vi "Teleop.vi"(10 "Match Info":T1={"Autonomous Elapsed Seconds"=0.0, "TeleOp Elapsed Seconds"=0.0, "Disabled Elapsed Seconds"=0.0, "Visited Autonomous"=FALSE, "Visited TeleOp"=FALSE, "Visited Disabled"=FALSE, "Autonomous Settings"={"Autonomous Style"=enum."Independent", "VI Refnum"=refnum}}, 11 "Call Context":T2) -> ()   [LabVIEW 2014]
doc: "This VI is called for each TeleOp packet received from the DS where the robot is not disabled. It is often used to read from the joysticks and update I/O or to update setpoints for timed control loops. It should complete and return within 20 milliseconds or it may miss DS packets."
uses:
  <vilib>/Rock Robotics/WPI/DriverStation/WPI_DriverStationDerivedRobotMode.ctl
  <vilib>/Rock Robotics/WPI/DriverStation/WPI_DriverStationMatch Info.ctl
  Robot Global Data.vi
  <vilib>/Rock Robotics/WPI/Joystick/WPI_JoystickGetSetRefNum.vi
  <vilib>/Rock Robotics/WPI/RobotDrive/WPI_RobotDriveGetSetRefNum.vi
panel:
  out "toggle on/off 2":bool=TRUE
  in  "toggle on/off internal 2":bool=TRUE
  in  "last switch 2":bool
  out "axis 1 (x) 2":dbl
  out "axis 2 (y) 2":dbl
  out "toggle on/off":bool=TRUE
  in  "toggle on/off internal":bool=TRUE
  in  "last switch":bool
  out "axis 1 (x)":dbl
  out "axis 2 (y)":dbl
  out "Numeric 1":dbl(slide) scale=0.0..100.0
  out "Boolean 2":bool
  out "Boolean 1":bool
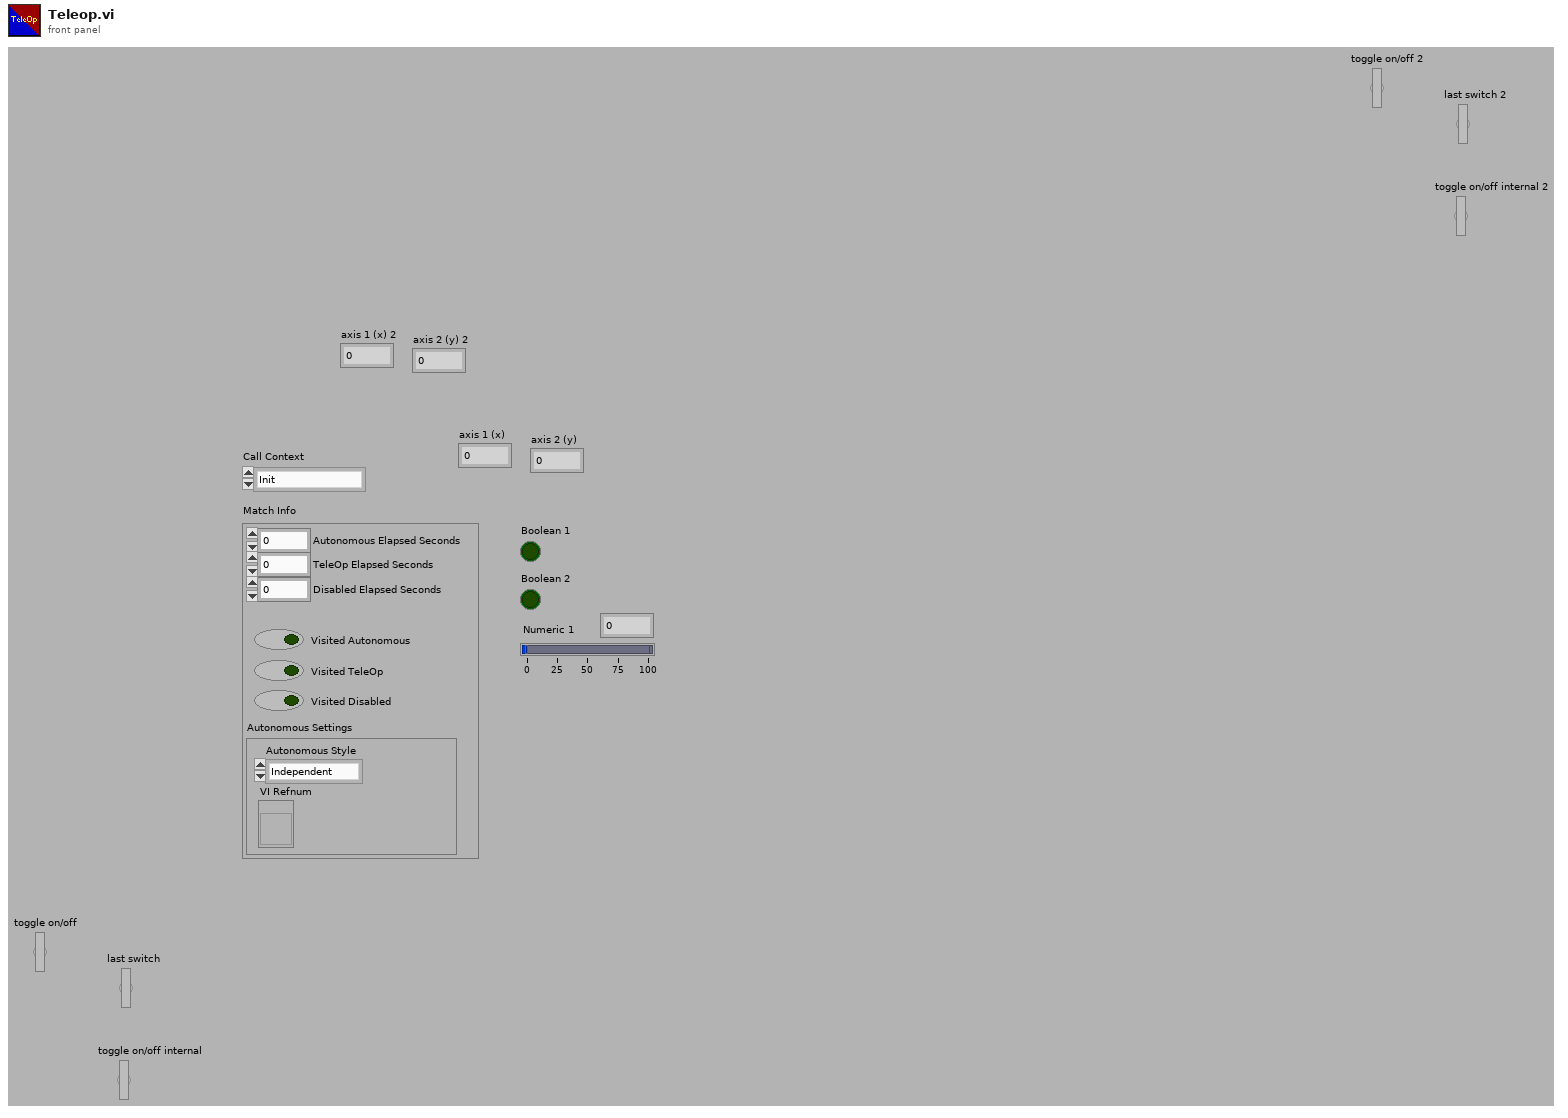
[diagram p1: front panel]
types:
  T1 = typedef "WPI_DriverStationMatch Info.ctl" = cluster{"Autonomous Elapsed Seconds":dbl, "TeleOp Elapsed Seconds":dbl, "Disabled Elapsed Seconds":dbl, "Visited Autonomous":bool, "Visited TeleOp":bool, "Visited Disabled":bool, "Autonomous Settings":cluster{"Autonomous Style":enum16{"Iterative", "Independent"}, "VI Refnum":refnum<vi>}}
  T2 = typedef "WPI_DriverStationDerivedRobotMode.ctl" = enum16{"Init", "Execute", "Stop"}
  T3 = typedef "WPI_JoystickDevRef.ctl" = cluster{"Device":T4}
  T4 = typedef "WPI_JoystickDeviceEnum.ctl" = enum16{"USB 0", "USB 1", "USB 2", "USB 3", "USB 4", "USB 5"}
  T5 = cluster{"Button 1":bool, "Button 2":bool, "Button 3":bool, "Button 4":bool, "Button 5":bool, "Button 6":bool, "Button 7":bool, "Button 8":bool, "Button 9":bool, "Button 10":bool, "Button 11":bool, "Button 12":bool}
  T6 = cluster{"axis 1 (x)":dbl, "axis 2 (y)":dbl, "axis 3 (throttle)":dbl, "axis 4":dbl, "axis 5":dbl, "axis 6":dbl}
  T7 = typedef "WPI_RobotDriveDevRef.ctl" = cluster{"DevStatus":errorcluster, "Motors[]":T8[], "Square Inputs":bool, "Max Output":dbl}
  T8 = typedef "WPI_MotorControlDeviceRef.ctl" = cluster{"DeviceStatus":errorcluster, "Type":enum16{"PWM", "CAN"}, "PWM":cluster{"Digital Module":T9, "PWM Channel":T10, "DeadBand":T11}, "CAN":cluster{"Device Number":u8, "Control Mode":T12, "Semaphore":T13, "Max Vout":dbl}, "Invert":bool, "TransformRef":T14, "InvTransformRef":T14}
  T9 = typedef "FPGA_TypedefDigitalModule.ctl" = enum16{"Digital Module 1", "Digital Module 2"}
  T10 = typedef "FPGA_DIOPWMChannel.ctl" = enum8{"PWM 1", "PWM 2", "PWM 3", "PWM 4", "PWM 5", "PWM 6", "PWM 7", "PWM 8", "PWM 9", "PWM 10", "Invalid"}
  T11 = typedef "WPI_PWMDeadband.ctl" = cluster{"Name":string, "maxPositivePwm":i32, "minPositivePwm":i32, "centerPwm":i32, "maxNegativePwm":i32, "minNegativePwm":i32, "angularRange":u16}
  T12 = typedef "WPI_CANJaguar_ControlMode.ctl" = enum8{"Percent VBus", "Current", "Speed", "Position", "Voltage"}
  T13 = typedef "Semaphore RefNum" = refnum<k1>
  T14 = typedef "WPI_PWMTransform_ConPane.ctl" = refnum<vi>
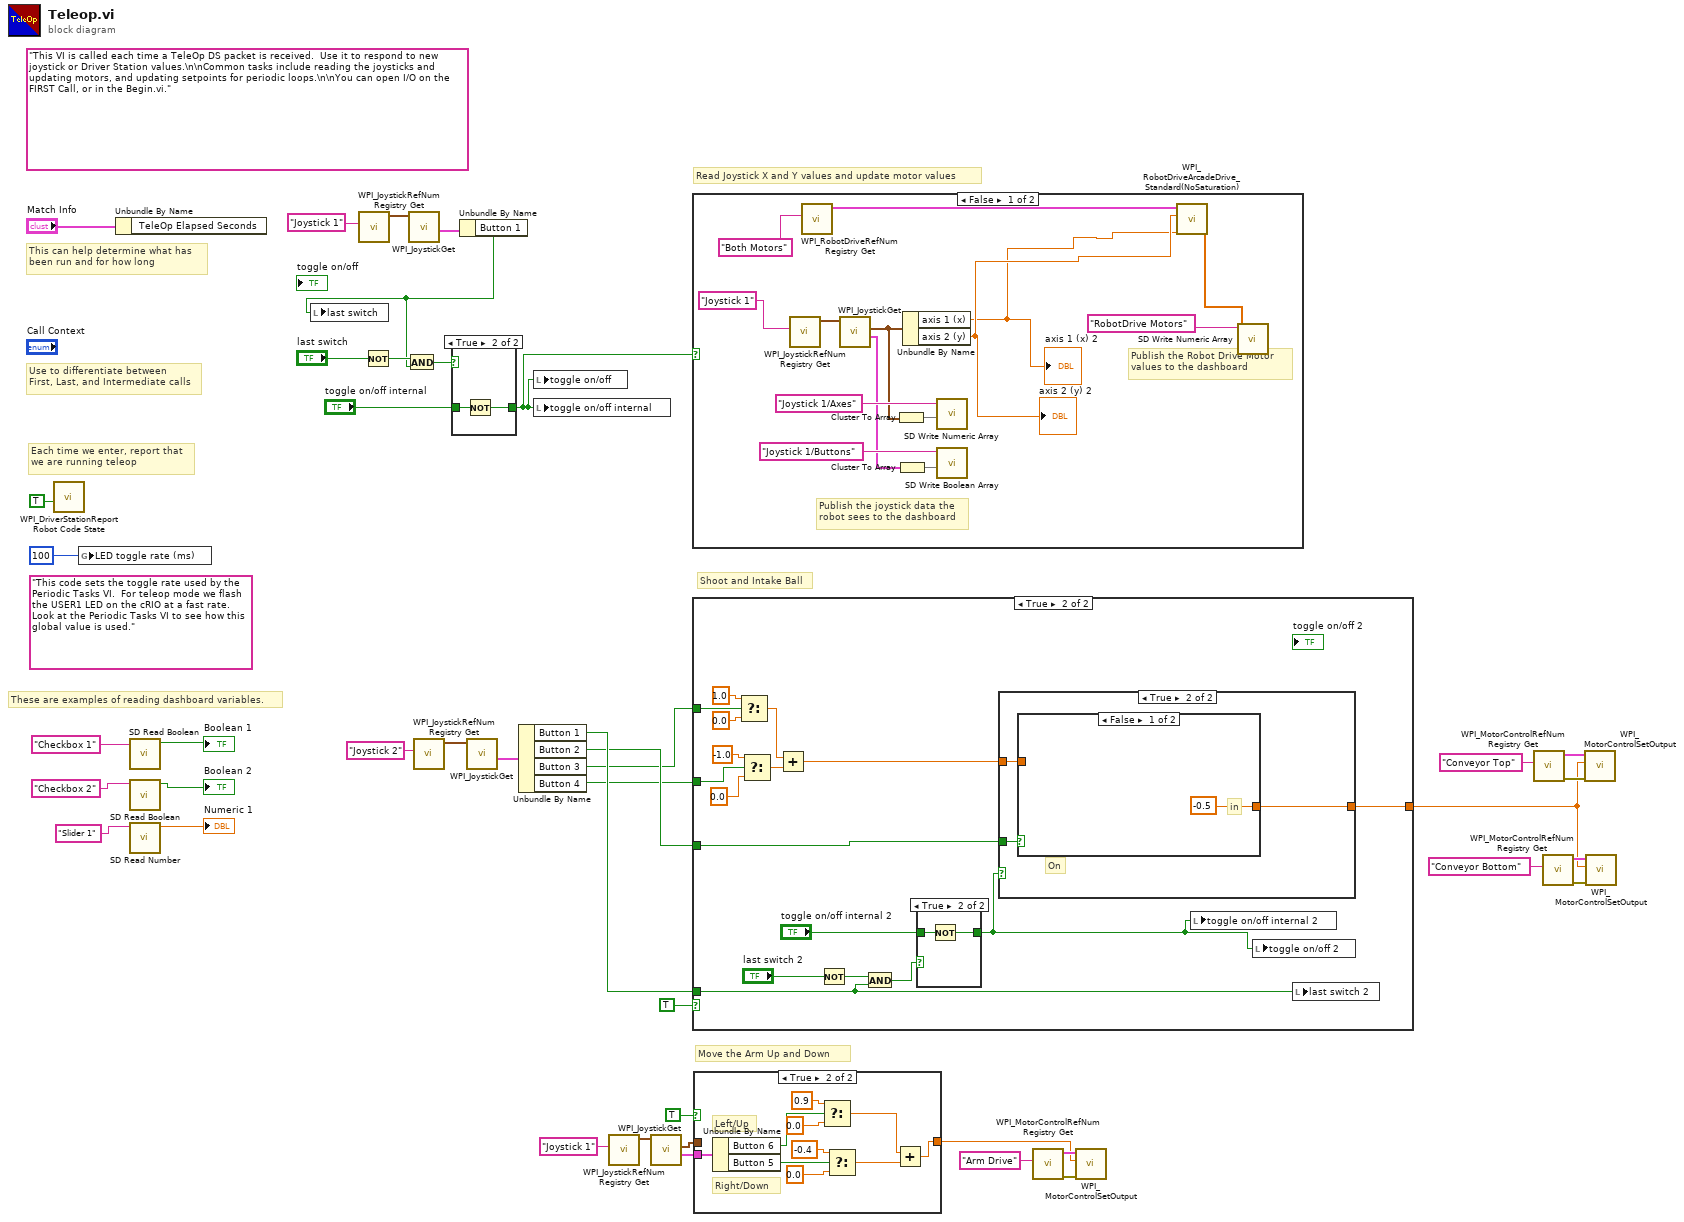
[diagram p0: block diagram]
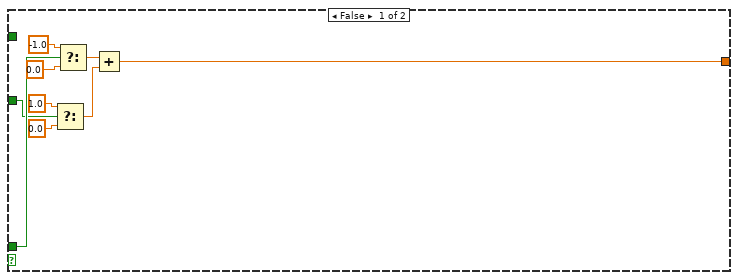
[diagram p2: hidden frame]
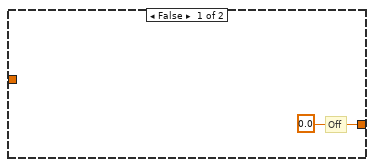
[diagram p4: hidden frame]
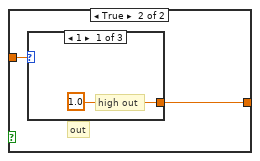
[diagram p5: hidden frame]
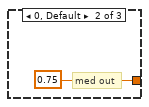
[diagram p6: hidden frame]
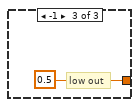
[diagram p7: hidden frame]
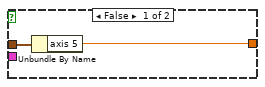
[diagram p8: hidden frame]
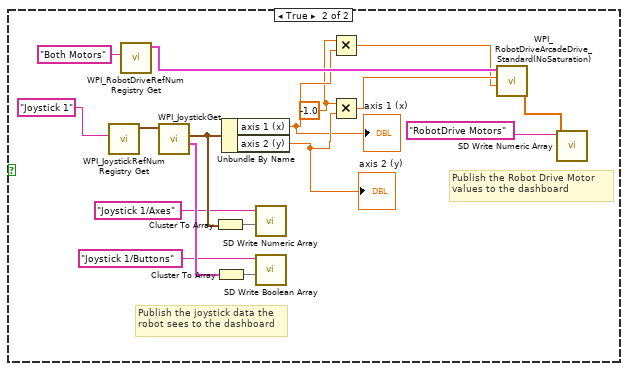
[diagram p10: hidden frame]
diagram:
  (unwired) "This code sets the toggle rate used by the Periodic Tasks VI.  For teleop mode we flash the USER1 LED on the cRIO at a fast rate.  Look at the Periodic Tasks VI to see how this global value is used."
  (unwired) "This VI is called each time a TeleOp DS packet is received.  Use it to respond to new joystick or Driver Station values.\n\nCommon tasks include reading the joysticks and updating motors, and updating setpoints for periodic loops.\n\nYou can open I/O on the FIRST Call, or in the Begin.vi."
  # "Move the Arm Up and Down"
  # "Shoot and Intake Ball"
  # "These are examples of reading dashboard variables."
  # "Each time we enter, report that\nwe are running teleop"
  # "Use to differentiate between\nFirst, Last, and Intermediate calls"
  # "This can help determine what has\nbeen run and for how long"
  # "Read Joystick X and Y values and update motor values"
  n1 = call <vilib>:"WPI_DriverStationReport Robot Code State.vi"("TeleOp"=TRUE ("Autonomous")) -> ()  [unwired: 10 in, 1 out]
  n2 = global write "Robot Global Data.vi" "LED toggle rate (ms)"(u32 100 ("LED ms toggle rate")) -> ()
  n3 = Unbundle By Name("Match Info") -> ()  [unwired: 1 out]
  n4 = call <vilib>:"SD Read Boolean.vi"("Name"="Checkbox 1" ("refnum name")) -> ("Boolean"=→"Boolean 1":bool)  [unwired: 8 in, 2 out]
  n5 = call <vilib>:"SD Read Boolean.vi"("Name"="Checkbox 2" ("refnum name")) -> ("Boolean"=→"Boolean 2":bool)  [unwired: 8 in, 2 out]
  n6 = call <vilib>:"SD Read Number.vi"("Name"="Slider 1" ("refnum name")) -> ("Numeric"=→"Numeric 1":dbl)  [unwired: 8 in, 2 out]
  n7 = call <vilib>:"WPI_JoystickRefNum Registry Get.vi"("refnum name"="Joystick 1") -> ("JoystickDevRef"=w17:T3)  [unwired: 1 in, 9 out]
  n8 = Not(x="last switch") -> (.not. x?=w13:bool)
  n9 = call <vilib>:"WPI_JoystickGet.vi"("JoystickDevRef"=w17) -> ("Buttons"=w15:T5)  [unwired: 1 in, 5 out]
  n10 = call <vilib>:"WPI_JoystickRefNum Registry Get.vi"("refnum name"="Joystick 2") -> ("JoystickDevRef"=w27:T3)  [unwired: 9 in, 1 out]
  n11 = Unbundle By Name(w15) -> ("Button 1"=w10:bool)
  n12 = local write "last switch"(w10) -> ()
  n13 = And(x=w13, y=w10) -> (x .and. y?=w12:bool)
  n14 = case shown="True" w12 {
    tunnel: "toggle on/off internal" -> [w43 w45]
    tunnel: [w43 w44] -> w1
    frame False {
    }
    frame True {
      n15 = Not(x=w45) -> (.not. x?=w44:bool)
    }
  }
  n16 = call <vilib>:"WPI_JoystickGet.vi"("JoystickDevRef"=w27) -> ("Buttons"=w25:T5)  [unwired: 4 in, 2 out]
  n17 = Unbundle By Name(w25) -> ("Button 1"=w9:bool, "Button 2"=w8:bool, "Button 3"=w7:bool, "Button 4"=w6:bool)
  n18 = local write "toggle on/off"(w1) -> ()
  n19 = local write "toggle on/off internal"(w1) -> ()
  n20 = call <vilib>:"WPI_JoystickRefNum Registry Get.vi"("refnum name"="Joystick 1") -> ("JoystickDevRef"=w32:T3)  [unwired: 9 in, 1 out]
  n21 = call <vilib>:"WPI_JoystickGet.vi"("JoystickDevRef"=w32) -> ("Buttons"=w31:T5, "Axes"=w3:T6)  [unwired: 4 in, 1 out]
  n22 = case shown="False" w1 {
    frame False {
      # "Publish the Robot Drive Motor\nvalues to the dashboard"
      # "Publish the joystick data the\nrobot sees to the dashboard"
      n23 = call <vilib>:"WPI_JoystickRefNum Registry Get.vi"("refnum name"="Joystick 1") -> ("JoystickDevRef"=w49:T3)  [unwired: 1 in, 9 out]
      n24 = call <vilib>:"WPI_RobotDriveRefNum Registry Get.vi"("refnum name"="Both Motors") -> ("RobotDriveDevRef"=w59:T7)  [unwired: 9 in, 1 out]
      n25 = call <vilib>:"WPI_JoystickGet.vi"("JoystickDevRef"=w49) -> ("Buttons"=w50:T5, "Axes"=w53:T6)  [unwired: 1 in, 4 out]
      n26 = Cluster To Array(cluster=w53) -> (array=w54:dbl[])
      n27 = Cluster To Array(cluster=w50) -> (array=w51:bool[])
      n28 = Unbundle By Name(w53) -> ("axis 1 (x)"=w46:dbl, "axis 2 (y)"=w47:dbl)
      "axis 2 (y) 2" <- w47
      "axis 1 (x) 2" <- w46
      n29 = call <vilib>:"SD Write Numeric Array.vi"("Numeric Array"=w54, "Name"="Joystick 1/Axes") -> ()  [unwired: 8 in, 2 out]
      n30 = call <vilib>:"SD Write Boolean Array.vi"("Boolean Array"=w51, "Name"="Joystick 1/Buttons") -> ()  [unwired: 8 in, 2 out]
      n31 = call <vilib>:"WPI_RobotDriveArcadeDrive_Standard(NoSaturation).vi"("Y axis value"=w46, "X axis value"=w47, "RobotDriveDevRef"=w59) -> ("Motor Values"=w57:dbl[])  [unwired: 1 in, 7 out]
      n32 = call <vilib>:"SD Write Numeric Array.vi"("Numeric Array"=w57, "Name"="RobotDrive Motors") -> ()  [unwired: 8 in, 2 out]
    }
    frame True {
      w60 = -1.0 ("x")
      # "Publish the Robot Drive Motor\nvalues to the dashboard"
      # "Publish the joystick data the\nrobot sees to the dashboard"
      n33 = call <vilib>:"WPI_JoystickRefNum Registry Get.vi"("refnum name"="Joystick 1") -> ("JoystickDevRef"=w75:T3)  [unwired: 1 in, 9 out]
      n34 = call <vilib>:"WPI_RobotDriveRefNum Registry Get.vi"("refnum name"="Both Motors") -> ("RobotDriveDevRef"=w65:T7)  [unwired: 9 in, 1 out]
      n35 = call <vilib>:"WPI_JoystickGet.vi"("JoystickDevRef"=w75) -> ("Buttons"=w74:T5, "Axes"=w71:T6)  [unwired: 1 in, 4 out]
      n36 = Cluster To Array(cluster=w71) -> (array=w70:dbl[])
      n37 = Cluster To Array(cluster=w74) -> (array=w73:bool[])
      n38 = Unbundle By Name(w71) -> ("axis 1 (x)"=w61:dbl, "axis 2 (y)"=w63:dbl)
      "axis 2 (y)" <- w63
      "axis 1 (x)" <- w61
      n39 = call <vilib>:"SD Write Numeric Array.vi"("Numeric Array"=w70, "Name"="Joystick 1/Axes") -> ()  [unwired: 8 in, 2 out]
      n40 = call <vilib>:"SD Write Boolean Array.vi"("Boolean Array"=w73, "Name"="Joystick 1/Buttons") -> ()  [unwired: 8 in, 2 out]
      n41 = Multiply(x=w60, y=w61) -> (x*y=w62:dbl)
      n42 = Multiply(x=w60, y=w63) -> (x*y=w64:dbl)
      n43 = call <vilib>:"WPI_RobotDriveArcadeDrive_Standard(NoSaturation).vi"("Y axis value"=w62, "X axis value"=w64, "RobotDriveDevRef"=w65) -> ("Motor Values"=w67:dbl[])  [unwired: 1 in, 7 out]
      n44 = call <vilib>:"SD Write Numeric Array.vi"("Numeric Array"=w67, "Name"="RobotDrive Motors") -> ()  [unwired: 8 in, 2 out]
    }
  }
  n45 = case shown="True" TRUE {
    tunnel: [w77 w102] -> w18
    tunnel: w9 -> [w84 w90]
    tunnel: w8 -> [w80 w88]
    tunnel: w7 -> [_ w87]
    tunnel: w6 -> [_ w86]
    frame False {
      n46 = Select(t=1.0, s=w80, f=0.0) -> (s? t:f=w78:dbl)
      n47 = Select(t=-1.0, s=w84, f=0.0) -> (s? t:f=w79:dbl)
      n48 = Add(x=w79, y=w78) -> (x+y=w77:dbl)
    }
    frame True {
      n49 = Select(t=1.0, s=w87, f=0.0) -> (s? t:f=w96:dbl)
      n50 = Select(t=-1.0, s=w86, f=0.0) -> (s? t:f=w97:dbl)
      n51 = Add(x=w96, y=w97) -> (x+y=w95:dbl)
      n52 = Not(x="last switch 2") -> (.not. x?=w93:bool)
      n53 = And(x=w93, y=w90) -> (x .and. y?=w92:bool)
      n54 = case shown="True" w92 {
        tunnel: "toggle on/off internal 2" -> [w103 w105]
        tunnel: [w103 w104] -> w89
        frame False {
        }
        frame True {
          n55 = Not(x=w105) -> (.not. x?=w104:bool)
        }
      }
      n56 = case shown="True" w89 {
        tunnel: [0.0 ("f") w108] -> w102
        tunnel: w95 -> [_ w109]
        tunnel: w88 -> [_ w107]
        frame False {
          # "Off"
        }
        frame True {
          # "On"
          n57 = case shown="False" w107 {
            tunnel: w109 -> [_ w112]
            tunnel: [-0.5 ("t") w111] -> w108
            frame False {
              # "in"
            }
            frame True {
              # "out"
              n58 = case shown="1" w112 {
                tunnel: [1.0 ("t") 0.75 ("t") 0.5 ("f")] -> w111
                frame 1 {
                  # "high out"
                }
                frame 0, Default {
                  # "med out"
                }
                frame -1 {
                  # "low out"
                }
              }
            }
          }
        }
      }
      n59 = local write "toggle on/off internal 2"(w89) -> ()
      n60 = local write "toggle on/off 2"(w89) -> ()
      n61 = local write "last switch 2"(w90) -> ()
    }
  }
  n62 = case shown="True" TRUE {
    tunnel: w31 -> [_ w127]
    tunnel: [w116 w118] -> w5
    tunnel: w3 -> [w117 _]
    frame False {
      n63 = Unbundle By Name(w117) -> ("axis 5"=w116:dbl)
    }
    frame True {
      # "Right/Down"
      # "Left/Up"
      n64 = Unbundle By Name(w127) -> ("Button 6"=w126:bool, "Button 5"=w125:bool)
      n65 = Select(t=0.9, s=w126, f=0.0) -> (s? t:f=w119:dbl)
      n66 = Select(t=-0.4, s=w125, f=0.0) -> (s? t:f=w120:dbl)
      n67 = Add(x=w119, y=w120) -> (x+y=w118:dbl)
    }
  }
  n68 = call <vilib>:"WPI_MotorControlRefNum Registry Get.vi"("refnum name"="Arm Drive") -> ("error out"=w30:errorcluster, "MotorControlDevRef"=w29:T8)  [unwired: 9 in]
  n69 = call <vilib>:"WPI_MotorControlSetOutput.vi"("error in (no error)"=w30, "Output"=w5, "MotorControlDevRef"=w29) -> ()  [unwired: 6 in, 3 out]
  n70 = call <vilib>:"WPI_MotorControlRefNum Registry Get.vi"("refnum name"="Conveyor Top") -> ("error out"=w22:errorcluster, "MotorControlDevRef"=w23:T8)  [unwired: 9 in]
  n71 = call <vilib>:"WPI_MotorControlRefNum Registry Get.vi"("refnum name"="Conveyor Bottom") -> ("error out"=w21:errorcluster, "MotorControlDevRef"=w20:T8)  [unwired: 9 in]
  n72 = call <vilib>:"WPI_MotorControlSetOutput.vi"("error in (no error)"=w22, "Output"=w18, "MotorControlDevRef"=w23) -> ()  [unwired: 6 in, 3 out]
  n73 = call <vilib>:"WPI_MotorControlSetOutput.vi"("error in (no error)"=w21, "Output"=w18, "MotorControlDevRef"=w20) -> ()  [unwired: 6 in, 3 out]
